vi "subFindAllSpecs.vi"(8 "error in (no error)":errorcluster, 11 "Project":path) -> (0 "error out":errorcluster, 2 "Build Specs":T1[](array[typedef]), 3 "dup Project":path)   [LabVIEW 2014, in "lvcommonbuild.lvlib"]
uses:
  lvcommonbuild.lvlib
  ctlTargetInfo.ctl
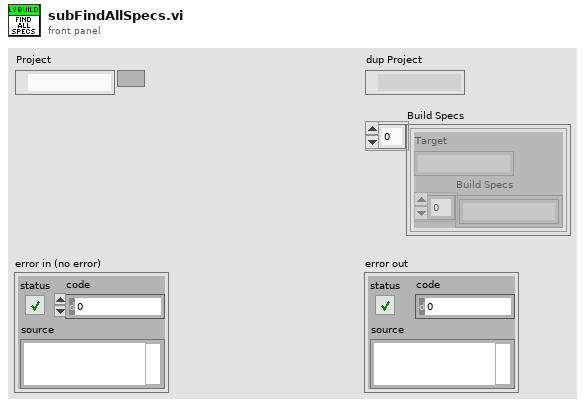
[diagram p1: front panel]
types:
  T1 = typedef "lvcommonbuild.lvlib/ctlTargetInfo.ctl" = cluster{"Target":string, "Build Specs":string[]}
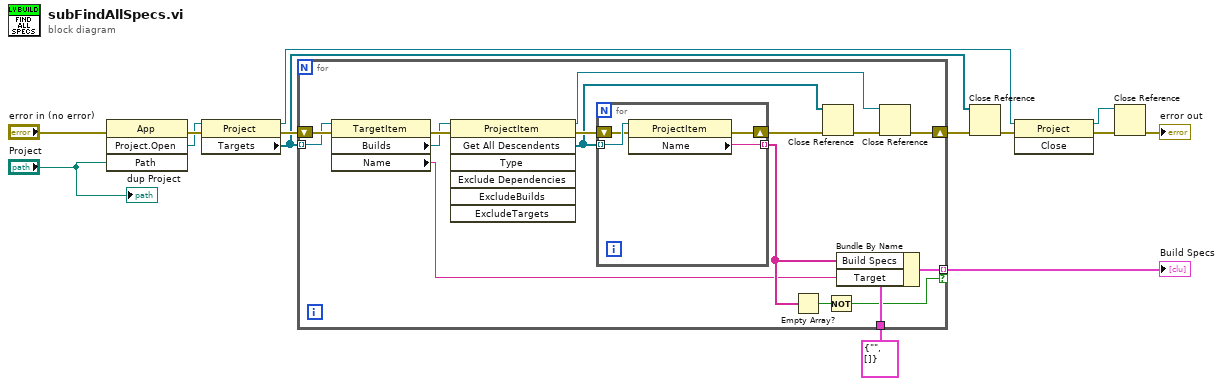
[diagram p0: block diagram]
diagram:
  n1 = invoke class="App" method="Project.Open"(error in="error in (no error)", "Path"="Project") -> (error out=w12:errorcluster, "Project:Open"=w11:refnum<vi>)  [unwired: 2 in, 2 out]
  n2 = property class="Project"(reference=w11, error in=w12) -> (reference out=w5:refnum<vi>, error out=w10:errorcluster, "Targets"=w7:refnum<vi>[])
  n3 = for {
    tunnel: w7 -> [w29] mode=indexing
    shift-right: [w22] -> w9
    shift-left: w10 -> [w30]
    tunnel: [w16] -> w1 mode=indexing if=w15
    tunnel: T1 {"Target"="", "Build Specs"=[]} ("Target Info") -> [w19]
    n4 = property class="TargetItem"(reference=w29, error in=w30) -> (error out=w28:errorcluster, "Builds"=w27:refnum<vi>, "Name"=w17:string)  [unwired: 1 out]
    n5 = invoke class="ProjectItem" method="Get All Descendents"(reference=w27, error in=w28) -> (reference out=w21:refnum<vi>, error out=w26:errorcluster, "All Descendents"=w23:refnum<vi>[])  [unwired: 5 in, 4 out]
    n6 = for {
      tunnel: w23 -> [w34] mode=indexing
      shift-right: [w32] -> w25
      shift-left: w26 -> [w33]
      tunnel: [w31] -> w18 mode=indexing
      n7 = property class="ProjectItem"(reference=w34, error in=w33) -> (error out=w32:errorcluster, "Name"=w31:string)  [unwired: 1 out]
    }
    n8 = Empty Array?(array=w18) -> (empty?=w20:bool)
    n9 = Close Reference(reference=w23, error in (no error)=w25) -> (error out=w24:errorcluster)
    n10 = Not(x=w20) -> (.not. x?=w15:bool)
    n11 = Bundle By Name(cluster=w19, "Build Specs"=w18, "Target"=w17) -> (w16:T1)
    n12 = Close Reference(reference=w21, error in (no error)=w24) -> (error out=w22:errorcluster)
  }
  "Build Specs" <- w1
  n13 = Close Reference(reference=w7, error in (no error)=w9) -> (error out=w8:errorcluster)
  n14 = invoke class="Project" method="Close"(reference=w5, error in=w8) -> (reference out=w3:refnum<vi>, error out=w6:errorcluster)  [unwired: 1 in, 1 out]
  n15 = Close Reference(reference=w3, error in (no error)=w6) -> (error out=→"error out":errorcluster)
  "dup Project" <- "Project"
